vi "get all paths.vi"(8 "error in (no error)":errorcluster, 10 "parent":string, 11 "JSON Value in":refnum<class "JSON Value.lvclass">) -> (0 "error out":errorcluster, 1 "Array":bool[](array[boolean]), 2 "paths":string[](array[string]))   [LabVIEW 2016, in "JSON Value.lvclass"]
uses:
  JSON Value.lvclass
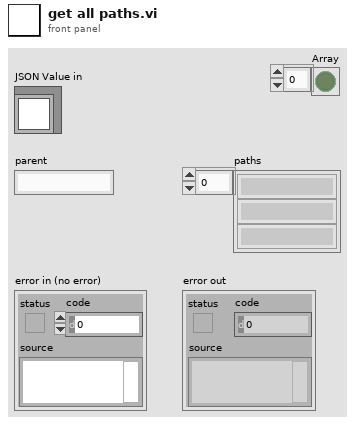
[diagram p1: front panel]
types:
  T1 = typedef "JSON Value.lvclass/JSON Types.ctl" = enum16{"String", "Numeric", "Boolean", "NULL", "Object", "Array"}
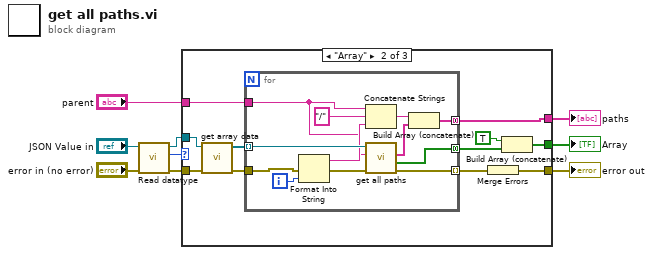
[diagram p0: block diagram]
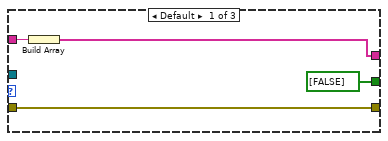
[diagram p2: hidden frame]
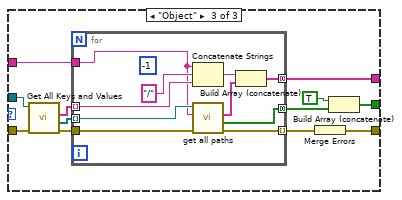
[diagram p3: hidden frame]
diagram:
  n1 = call "Read datatype.vi"("error in (no error)"="error in (no error)", "JSON Value in"="JSON Value in") -> ("error out"=w9:errorcluster, "datatype"=w5:T1, "JSON Value out"=w6:refnum<class "JSON Value.lvclass">)  [unwired: 7 in]
  n2 = case shown="\"Array\"" w5 {
    tunnel: [w10 w17 w37] -> w3
    tunnel: w9 -> [w13 w15 w43]
    tunnel: [w13 w23 w47] -> w1
    tunnel: [bool[] [FALSE] w21 w45] -> w7
    tunnel: w6 -> [_ w19 w42]
    tunnel: "parent" -> [w11 w16 w38]
    frame Default {
      n3 = Build Array(w11) -> (w10:string[])
    }
    frame "Array" {
      n4 = call "get array data.vi"("error in (no error)"=w15, "JSON Value in"=w19) -> ("error out"=w14:errorcluster, "JSON Array out"=w18:refnum<class "JSON Value.lvclass">[])  [unwired: 8 in]
      n5 = for {
        tunnel: [w36] -> w24 mode=indexing
        tunnel: [w35] -> w20 mode=concatenating
        tunnel: w18 -> [w34] mode=indexing
        tunnel: [w28] -> w17 mode=concatenating
        tunnel: w16 -> [w25]
        tunnel: w14 -> [w27]
        i -> [w31]
        n6 = Format Into String(error in=w27, w31) -> (resulting string=w32:string, error out=w26:errorcluster)  [unwired: 2 in]
        n7 = Concatenate Strings(w25, "/" ("string"), w32) -> (w30:string)
        n8 = call "get all paths.vi"("error in (no error)"=w26, "parent"=w25, "JSON Value in"=w34) -> ("error out"=w36:errorcluster, "Array"=w35:bool[], "paths"=w29:string[])  [unwired: 6 in]
        n9 = Build Array (concatenate)(w30, w29) -> (w28:string[])
      }
      n10 = Merge Errors(w24) -> (w23:errorcluster)
      n11 = Build Array (concatenate)(TRUE ("Boolean"), w20) -> (w21:bool[])
    }
    frame "Object" {
      n12 = call "Get All Keys and Values.vi"("error in"=w43, "JSON Value in"=w42) -> ("error out"=w41:errorcluster, "values"=w40:refnum<class "JSON Value.lvclass">[], "keys"=w39:string[])  [unwired: 7 in]
      n13 = for {
        tunnel: w41 -> [w58]
        tunnel: [w57] -> w48 mode=indexing
        tunnel: [w56] -> w44 mode=concatenating
        tunnel: w40 -> [w55] mode=indexing
        tunnel: w39 -> [w53] mode=indexing
        tunnel: w38 -> [w49]
        tunnel: [w50] -> w37 mode=concatenating
        (unwired) -1 ("index")
        n14 = Concatenate Strings(w49, "/" ("string"), w53) -> (w52:string)
        n15 = call "get all paths.vi"("error in (no error)"=w58, "parent"=w49, "JSON Value in"=w55) -> ("error out"=w57:errorcluster, "Array"=w56:bool[], "paths"=w51:string[])  [unwired: 6 in]
        n16 = Build Array (concatenate)(w52, w51) -> (w50:string[])
      }
      n17 = Merge Errors(w48) -> (w47:errorcluster)
      n18 = Build Array (concatenate)(TRUE, w44) -> (w45:bool[])
    }
  }
  "error out" <- w1
  "paths" <- w3
  "Array" <- w7
